vi "ListAllReposBranches.vi"(8 "error in (no error)":errorcluster, 11 "CommandLine":string[](array[string])) -> (0 "error out":errorcluster, 2 "test details":string)   [LabVIEW 2019]
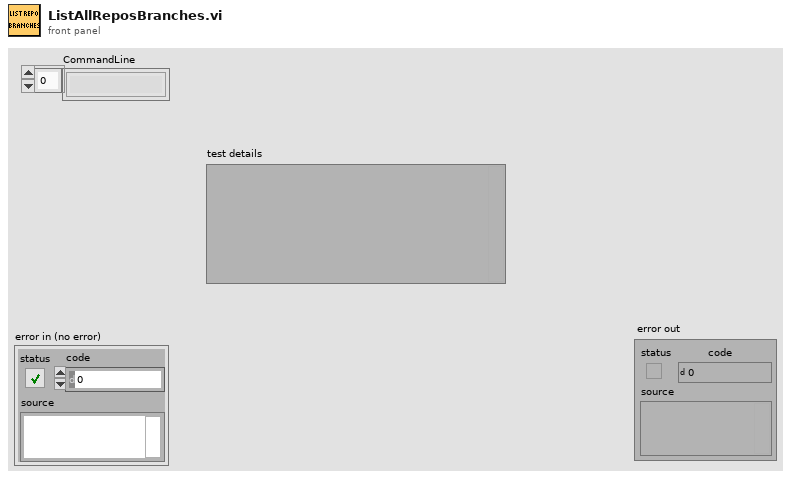
[diagram p1: front panel]
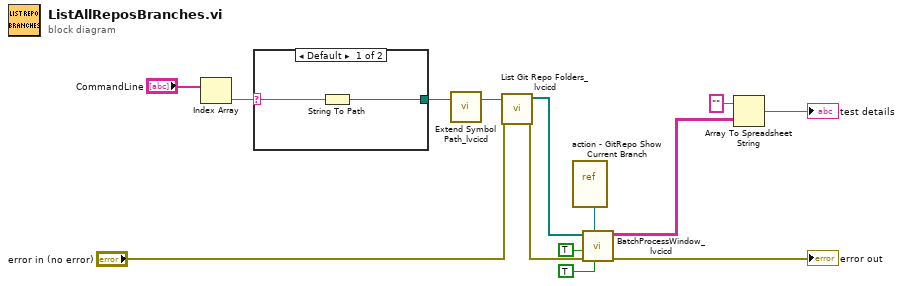
[diagram p0: block diagram]
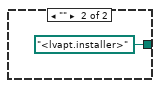
[diagram p2: hidden frame]
diagram:
  n1 = Index Array(array="CommandLine") -> (element=w1:string)  [unwired: 1 in]
  n2 = case shown="Default" w1 {
    selector: w1 -> [w16 _]
    tunnel: [w15 path "<lvapt.installer>"] -> w8
    frame Default {
      n3 = String To Path(string=w16) -> (path=w15:path)
    }
    frame "" {
    }
  }
  n4 = call "Extend Symbol Path_lvcicd.vi"("Symbol Path"=w8) -> ("Resolved Path"=w6:path)  [unwired: 2 in]
  n5 = call "List Git Repo Folders_lvcicd.vi"("error in (no error)"="error in (no error)", "path"=w6) -> ("error out"=w5:errorcluster, "Repo Folders"=w13:path[])  [unwired: 8 in]
  n6 = vi-ref "action - GitRepo Show Current Branch.vi"() -> (w7:refnum<vi>)
  n7 = call "BatchProcessWindow_lvcicd.vi"("FP(T)"=TRUE, "VI Refnum"=w7, "error in (no error)"=w5, "silence mode(F)"=TRUE, "paths"=w13) -> ("error out"=→"error out":errorcluster, "Array"=w12:string[][])  [unwired: 5 in]
  n8 = Array To Spreadsheet String(array=w12, 3:"" ("format string")) -> (spreadsheet string=→"test details":string)  [unwired: 1 in]
